vi "1 Channel 1 Sample - Auto Indexing.vi"() -> ()   [LabVIEW 2026]
uses:
  <userlib>/Synnax/synnax_lib.lvlibp/typedefs/connection_config.ctl
  <userlib>/Synnax/synnax_lib.lvlibp/classes/Client/Private/synnax channel retrieve keys Single.vi
  <userlib>/Synnax/synnax_lib.lvlibp/classes/Writer/Private/synnax writer open Single.vi
  <userlib>/Synnax/synnax_lib.lvlibp/classes/Writer/Private/Writes/String/Write 1Ch 1Samp (String).vi
  <userlib>/Synnax/synnax_lib.lvlibp/classes/Client/Synnax Client.lvclass
  <userlib>/Synnax/synnax_lib.lvlibp/classes/Synnax Writer.lvclass
  <userlib>/Synnax/synnax_lib.lvlibp
panel:
  in  "Connection Config":T1={"host"="localhost", "port"=9090, "username"="synnax", "password"="seldon"}
  in  "Edit Me:":string="This is \na multiline string\nthat I wrote \nto test writing to string channels"
  in  "Channel":string="my_str_chan"
  out "error out":errorcluster
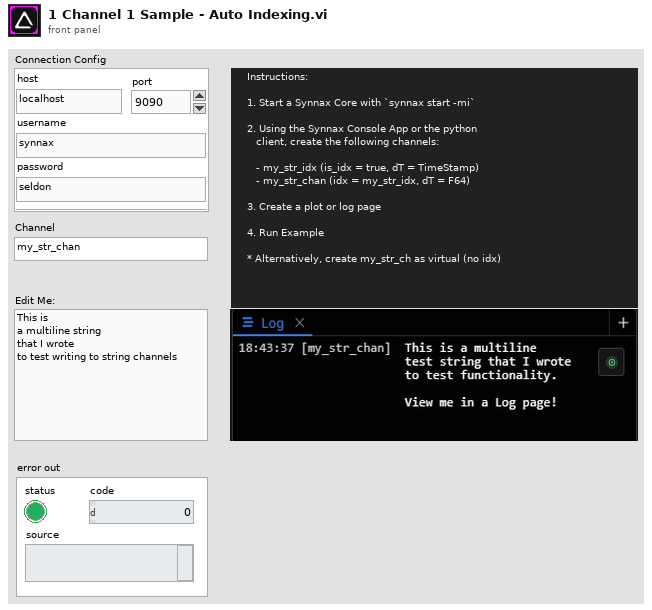
[diagram p1: front panel]
types:
  T1 = typedef "synnax_lib.lvlibp/connection_config.ctl" = cluster{"host":string, "port":u16, "username":string, "password":string}
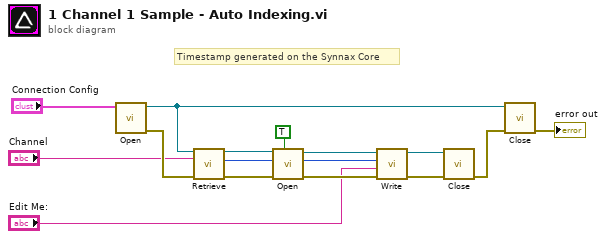
[diagram p0: block diagram]
diagram:
  # "Timestamp generated on the Synnax Core"
  n1 = call <userlib>:"Open.vi"("Connection Config"="Connection Config") -> ("error out"=w12:errorcluster, "Synnax Client out"=w14:refnum<class "Synnax Client.lvclass">)  [unwired: 9 in]
  n2 = call-poly <userlib>:"Retrieve.vi"("Synnax Client in"=w14, "channel name"="Channel", "error in"=w12) -> ("Synnax Client out"=w8:refnum<class "Synnax Client.lvclass">, "channel key"=w5:u32, "error out"=w15:errorcluster)  [unwired: 8 in, 2 out]
  n3 = call-poly <userlib>:"Open.vi"("auto_index (F)"=TRUE, "error in"=w15, "channel in"=w5, "Synnax Client in"=w8) -> ("error out"=w9:errorcluster, "channel out"=w6:u32, "writer out"=w11:refnum<class "Synnax Writer.lvclass">)  [unwired: 5 in]
  n4 = call-poly <userlib>:"Write.vi"("error in"=w9, "data"="Edit Me:", "channel"=w6, "Writer"=w11) -> ("error out"=w16:errorcluster, "Writer Out"=w10:refnum<class "Synnax Writer.lvclass">)  [unwired: 6 in]
  n5 = call <userlib>:"Close.vi"("error in"=w16, "writer"=w10) -> ("error out"=w13:errorcluster)  [unwired: 9 in]
  n6 = call <userlib>:"Close.vi"("error in"=w13, "Synnax Client in"=w14) -> ("error out"=→"error out":errorcluster)  [unwired: 9 in]
